vi "example1_leds.vi"() -> ()   [LabVIEW 2017]
uses:
  <vilib>/Stratom, Inc/X-CAN for myRIO (API)/X-CAN Class/Type Definitions/CAN_Speed.ctl
  <vilib>/Stratom, Inc/X-Modules for myRIO/Type Defs/MXPChannel.ctl
  <vilib>/Stratom, Inc/X-CAN for myRIO (API)/X-CAN Class/Type Definitions/CANFrame.ctl
  <vilib>/Stratom, Inc/X-CAN for myRIO (API)/X-CAN Class/X-CAN.lvclass
panel:
  out "pack sum voltage":dbl
  out "Battery Current":dbl
  out "supply voltage":dbl
  out "payload[3]":u8 format="%x"
  out "payload[2]":u8 format="%x"
  out "payload[1]":u8 format="%x"
  out "payload[0]":u8
  out "CAN Frame":T1 {"payload" format="%x"; "timestamp" format="%<%I:%M:%S%8u %p\n%x>T"; "identifier" format="%x"}
  in  "CAN Frame 2":T1 {"payload" format="%x"; "timestamp" format="%<%I:%M:%S%8u %p\n%x>T"; "identifier" format="%x"}
  in  "milliseconds to wait":u32
  in  "Numeric":i32
  in  "MXP Channel":T2
  in  "CAN Speed [Kbps]":T3 items=["125 Kbps"=7, "250 Kbps"=3, "500 Kbps"=1, "1000 Kbps"=0, "95.238 Kbps"=6]
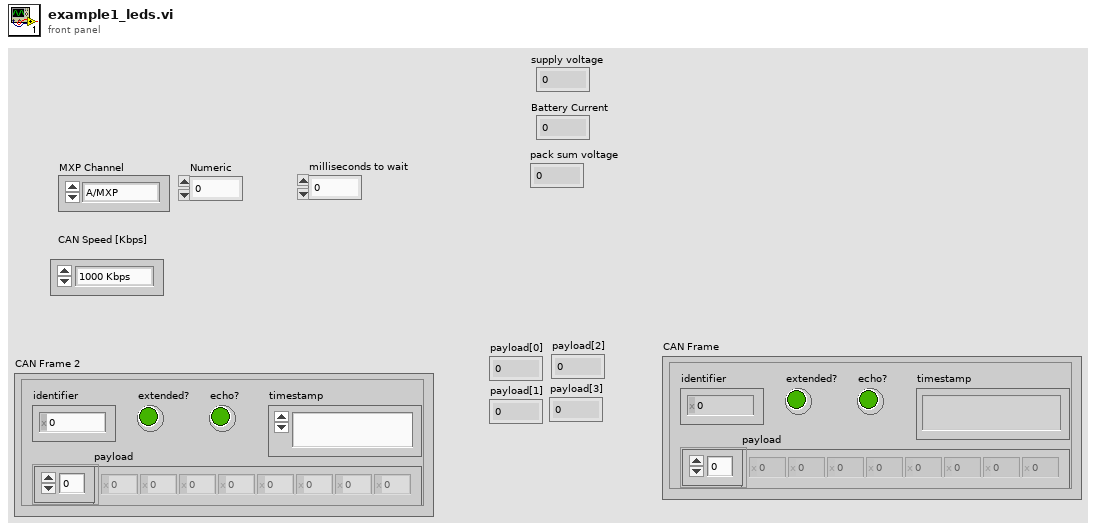
[diagram p1: front panel]
types:
  T1 = typedef "X-CAN.lvclass/CANFrame.ctl" = cluster{"identifier":u32, "extended?":bool, "echo?":bool, "payload":u8[], "timestamp":timestamp}
  T2 = typedef "MXPChannel.ctl" = enum16{"A/MXP", "B/MXP"}
  T3 = typedef "X-CAN.lvclass/CAN_Speed.ctl" = u8
  T4 = cluster{"payload[0]":u8, "payload[1]":u8, "payload[2]":u8, "payload[3]":u8, "payload[4]":u8, "payload[5]":u8, "payload[6]":u8, "payload[7]":u8, "payload[8]":u8}
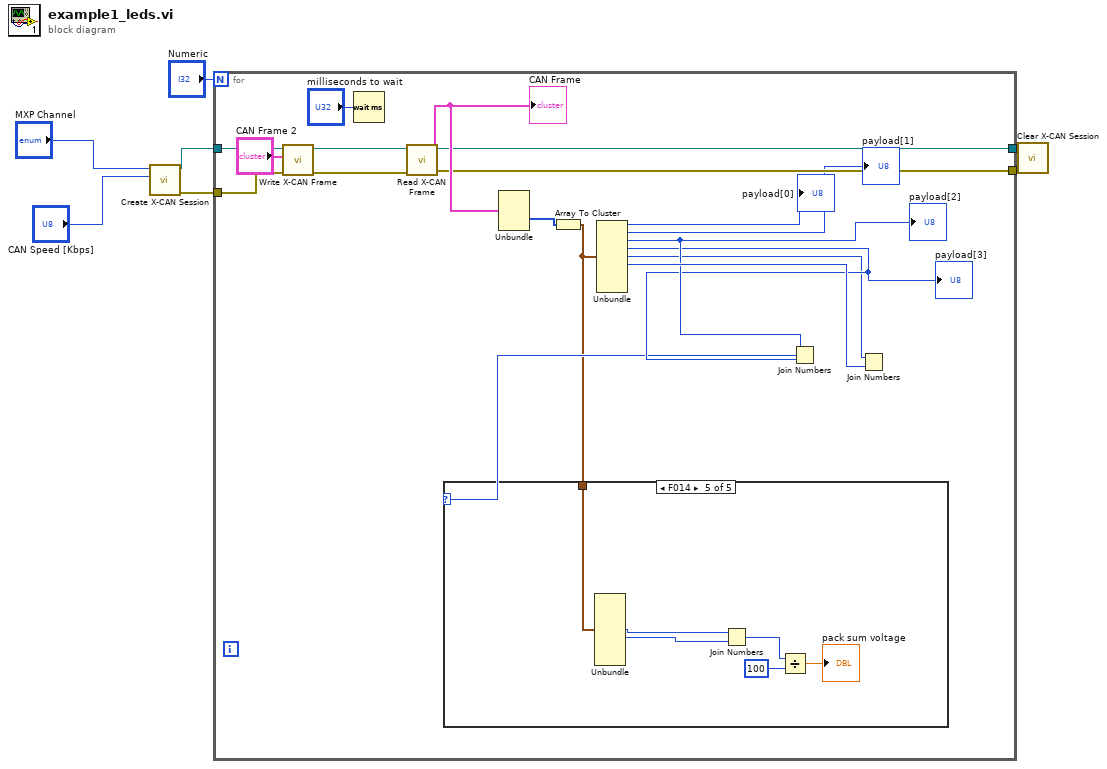
[diagram p0: block diagram]
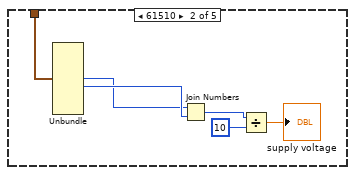
[diagram p3: hidden frame]
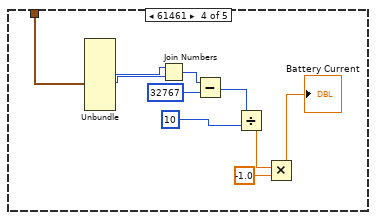
[diagram p5: hidden frame]
diagram:
  n1 = call <vilib>:"Create X-CAN Session.vi"("CAN Speed [Kbps]"="CAN Speed [Kbps]", "MXP Channel"="MXP Channel") -> ("error out"=w4:errorcluster, "X-CAN Session out"=w3:refnum<class "X-CAN.lvclass">)  [unwired: 8 in]
  n2 = for {
    N: "Numeric" -> [_]
    tunnel: w3 -> [w24]
    tunnel: w4 -> [w22]
    tunnel: [w18] -> w2
    tunnel: [w17] -> w1
    n3 = call <vilib>:"Write X-CAN Frame.vi"("error in"=w22, "CAN Frame"="CAN Frame 2", "X-CAN Session in"=w24) -> ("error out"=w21:errorcluster, "X-CAN Session out"=w23:refnum<class "X-CAN.lvclass">)  [unwired: 7 in]
    n4 = Wait (ms)(milliseconds to wait="milliseconds to wait") -> ()  [unwired: 1 out]
    n5 = call <vilib>:"Read X-CAN Frame.vi"("error in"=w21, "X-CAN Session in"=w23) -> ("error out"=w17:errorcluster, "CAN Frame"=w19:T1, "X-CAN Session out"=w18:refnum<class "X-CAN.lvclass">)  [unwired: 7 in]
    "CAN Frame" <- w19
    n6 = Unbundle(w19) -> ("payload"=w16:u8[])  [unwired: 4 out]
    n7 = Array To Cluster(array=w16) -> (cluster=w9:T4)
    n8 = Unbundle(w9) -> ("payload[0]"=→"payload[0]":u8, "payload[1]"=→"payload[1]":u8, "payload[2]"=w12:u8, "payload[3]"=w11:u8, "payload[4]"=w8:u8, "payload[5]"=w13:u8)  [unwired: 3 out]
    "payload[2]" <- w12
    "payload[3]" <- w11
    n9 = Join Numbers(hi=w12, lo=w11) -> ((hi.lo)=w10:u16)
    n10 = case shown="F014" w10 {
      tunnel: w9 -> [_ w31 _ w40 w47]
      frame 0, Default {
      }
      frame 61510 {
        n11 = Unbundle(w31) -> ("payload[4]"=w29:u8, "payload[5]"=w30:u8)  [unwired: 7 out]
        n12 = Join Numbers(hi=w29, lo=w30) -> ((hi.lo)=w28:u16)
        n13 = Divide(x=w28, y=u16 10) -> (x/y=→"supply voltage":dbl)
      }
      frame 2 {
      }
      frame 61461 {
        n14 = Unbundle(w40) -> ("payload[4]"=w39:u8, "payload[5]"=w38:u8)  [unwired: 7 out]
        n15 = Join Numbers(hi=w39, lo=w38) -> ((hi.lo)=w37:u16)
        n16 = Subtract(x=w37, y=u16 32767) -> (x-y=w35:u16)
        n17 = Divide(x=w35, y=u16 10) -> (x/y=w33:dbl)
        n18 = Multiply(x=w33, y=-1.0) -> (x*y=→"Battery Current":dbl)
      }
      frame 61460 {
        n19 = Unbundle(w47) -> ("payload[4]"=w45:u8, "payload[5]"=w46:u8)  [unwired: 7 out]
        n20 = Join Numbers(hi=w45, lo=w46) -> ((hi.lo)=w44:u16)
        n21 = Divide(x=w44, y=u16 100) -> (x/y=→"pack sum voltage":dbl)
      }
    }
    n22 = Join Numbers(hi=w8, lo=w13) -> ()  [unwired: 1 out]
  }
  n23 = call <vilib>:"Clear X-CAN Session.vi"("error in (no error)"=w1, "X-CAN Session in"=w2) -> ()  [unwired: 9 in, 1 out]
